vi "Load Transient.vi"() -> ()   [LabVIEW 2021]
uses:
  pmbus_ltm4676a/controls/ltm4676a_config.ctl
  controls/lt_nightwing_config.ctl
  controls/lt_heatwave_config.ctl
  controls/lt_system_timing_config.ctl
  <instrlib>/niDCPower/nidcpower.llb/niDCPower Source Mode.ctl
  <instrlib>/niDCPower/nidcpower.llb/niDCPower Output Function.ctl
  <instrlib>/niDCPower/nidcpower.llb/niDCPower Sense.ctl
  <instrlib>/niDCPower/nidcpower.llb/niDCPower Wait For Event - Event.ctl
  <instrlib>/niDCPower/nidcpower.llb/niDCPower Aperture Time Units.ctl
  <instrlib>/niDCPower/nidcpower.llb/niDCPower Export Signal - Signal.ctl
  <instrlib>/niDCPower/nidcpower.llb/niDCPower Disable Source Trigger With Channels.vi
panel:
  in  "App control":enum32{"Main", "Debug"}(tab)
  out "Load Transient Response":T1
  in  "Config control":T2(tab)
  in  "Source config":T3={"Source device name"="PXIe-4151", "Source device channel"="0", "Source device max. power (W)"=300.0, "Source device voltage (V)"=12.0, "Voltage GBW (Hz)"=2000.0, "Voltage comp. freq. (Hz)"=3530.0, "Voltage PZ ratio"=2.0}
  in  "Load config":T4={"Load device name"="PXIe-4051", "Load device channel"="0", "Load voltage limit (V)"=6.0, "Load device sample rate (S/s)"=1800000.0, "Current Setpoints"=[1.0, 20.0, 1.0], "Current GBW (Hz)"=14000.0, "Current comp. freq. (Hz)"=180000.0, "Current PZ ratio"=0.3} {"Current PZ ratio" min=0.0 max=8.0 step=0.1; "Current GBW (Hz)" min=0.0 step=1000.0; "Current Setpoints" format="%.2p"}
  in  "System timing config":T5={"DUT setup time (s)"=1.0, "Level dwell time (s)"=0.001, "Timeout (s)"=5.0} {"Timeout (s)" format="%.3p"; "Level dwell time (s)" step=0.0001; "DUT setup time (s)" format="%_4p"}
  in  "LTM4676A Runtime Config":T6={"SDC config path"=path "C:/dev/users/qkocian/opp_support/demos/argus-buck-demo/instrumentstudio/sdc/pmbus_ltm4676a.sdconfig", "Output setpoint (V)"=3.3, "Voltage margin (%)"=5.0, "Voltage warn limit (%)"=7.5, "Voltage fault limit (%)"=10.0, "Switching frequency (kHz)"=650} {"Switching frequency (kHz)" items=["250"=62440, "350"=64188, "425"=64338, "500"=64488, "575"=575, "650"=650, "750"=750, "1000"=1000]; "Voltage fault limit (%)" min=0.0 max=100.0 step=1.0 format="%.1g"; "Voltage warn limit (%)" min=0.0 max=100.0 step=1.0 format="%.1g"; "Voltage margin (%)" min=0.0 max=100.0 step=1.0 format="%.1g"; "Output setpoint (V)" min=0.5 max=5.5 step=0.1}
  in  "stop":bool
  out "success?":bool
  out "Current GBW readback (Hz)":dbl
  out "Current comp. freq. readback (Hz)":dbl
  out "Current PZ ratio readback":dbl
  in  "Waveform averages":i32=1
  out "Voltage GBW readback (Hz)":dbl
  out "Voltage comp. freq. readback (Hz)":dbl
  out "Voltage PZ ratio readback":dbl
  in  "Use PMBus?":bool
  # "Load SourceAdapt Readback"
  # "Source SourceAdapt Readback"
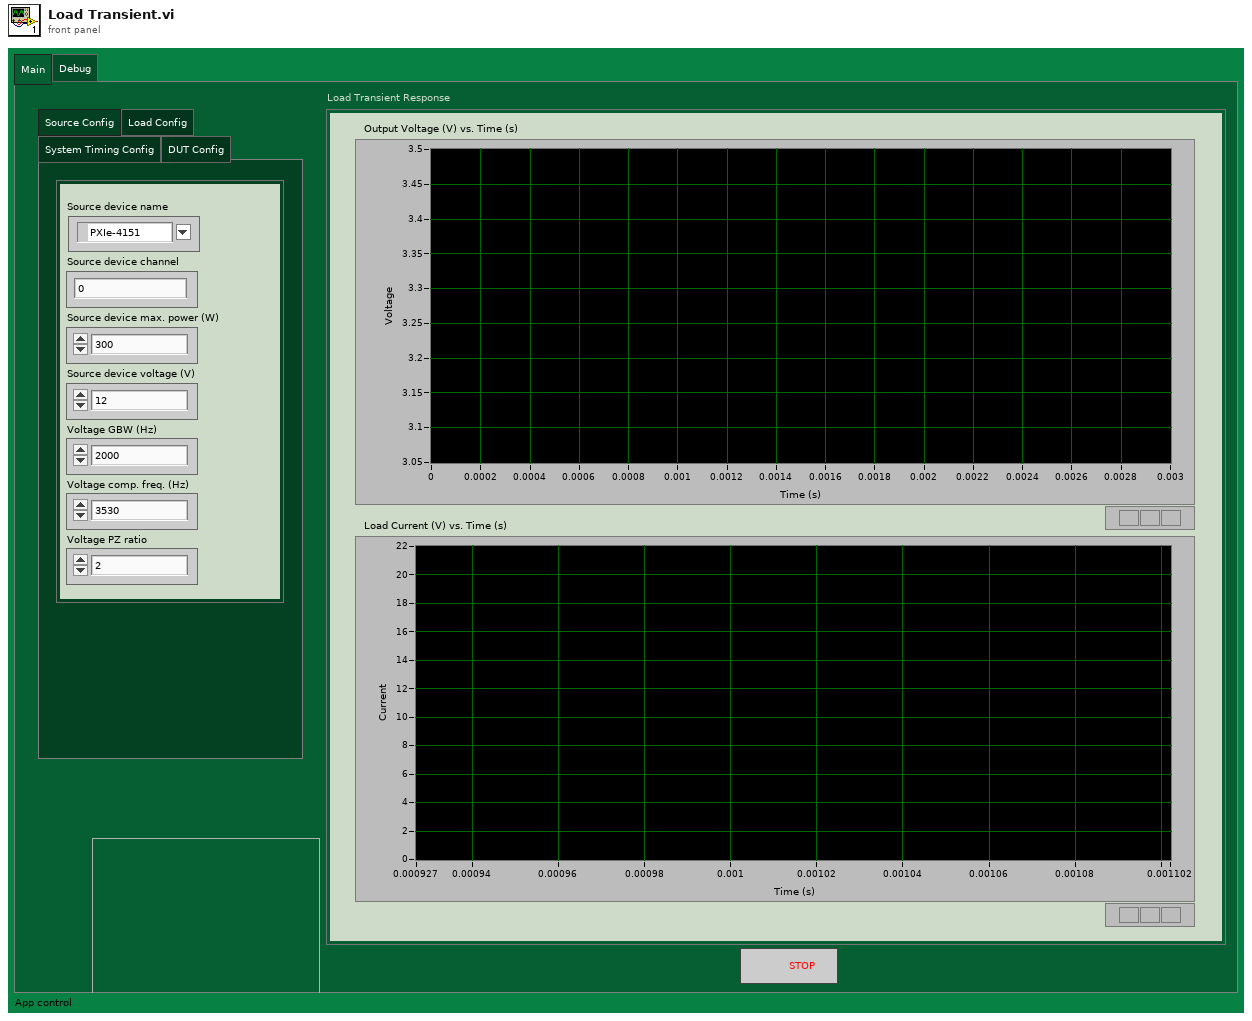
[diagram p1: front panel]
types:
  T1 = cluster{"Output Voltage (V) vs. Time (s)":waveform(dbl), "Load Current (V) vs. Time (s)":waveform(dbl)}
  T2 = enum32{"Source Config", "Load Config", "System Timing Config", "DUT Config"}
  T3 = typedef "lt_nightwing_config.ctl" = cluster{"Source device name":refnum<k15>, "Source device channel":string, "Source device max. power (W)":dbl, "Source device voltage (V)":dbl, "Voltage GBW (Hz)":dbl, "Voltage comp. freq. (Hz)":dbl, "Voltage PZ ratio":dbl}
  T4 = typedef "lt_heatwave_config.ctl" = cluster{"Load device name":refnum<k15>, "Load device channel":string, "Load voltage limit (V)":dbl, "Load device sample rate (S/s)":dbl, "Current Setpoints":dbl[], "Current GBW (Hz)":dbl, "Current comp. freq. (Hz)":dbl, "Current PZ ratio":dbl}
  T5 = typedef "lt_system_timing_config.ctl" = cluster{"DUT setup time (s)":dbl, "Level dwell time (s)":dbl, "Timeout (s)":dbl}
  T6 = typedef "ltm4676a_config.ctl" = cluster{"SDC config path":path, "Output setpoint (V)":dbl, "Voltage margin (%)":dbl, "Voltage warn limit (%)":dbl, "Voltage fault limit (%)":dbl, "Switching frequency (kHz)":u16}
  T7 = typedef "niDCPower Sense.ctl" = i32
  T8 = typedef "niDCPower Output Function.ctl" = i32
  T9 = typedef "niDCPower Source Mode.ctl" = i32
  T10 = typedef "niDCPower Wait For Event - Event.ctl" = i32
  T11 = typedef "niDCPower Export Signal - Signal.ctl" = i32
  T12 = typedef "niDCPower Aperture Time Units.ctl" = i32
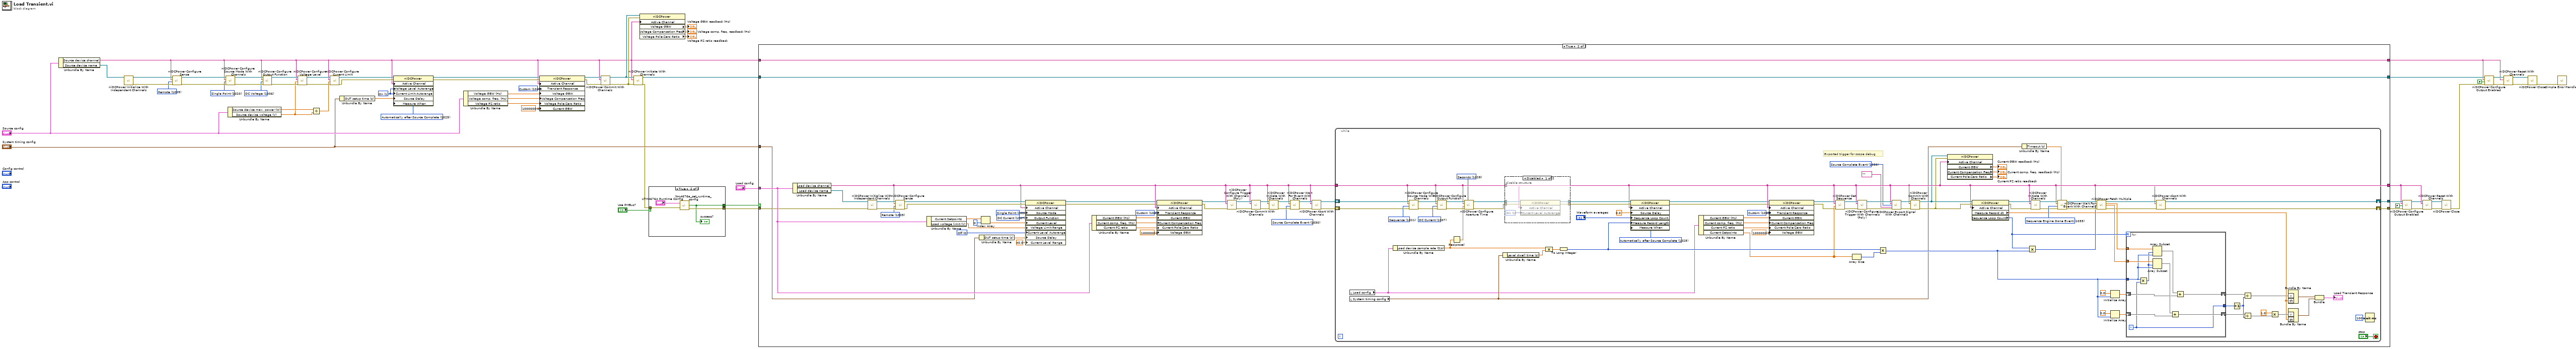
[diagram p0: block diagram]
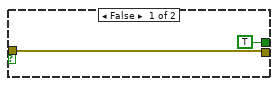
[diagram p2: hidden frame]
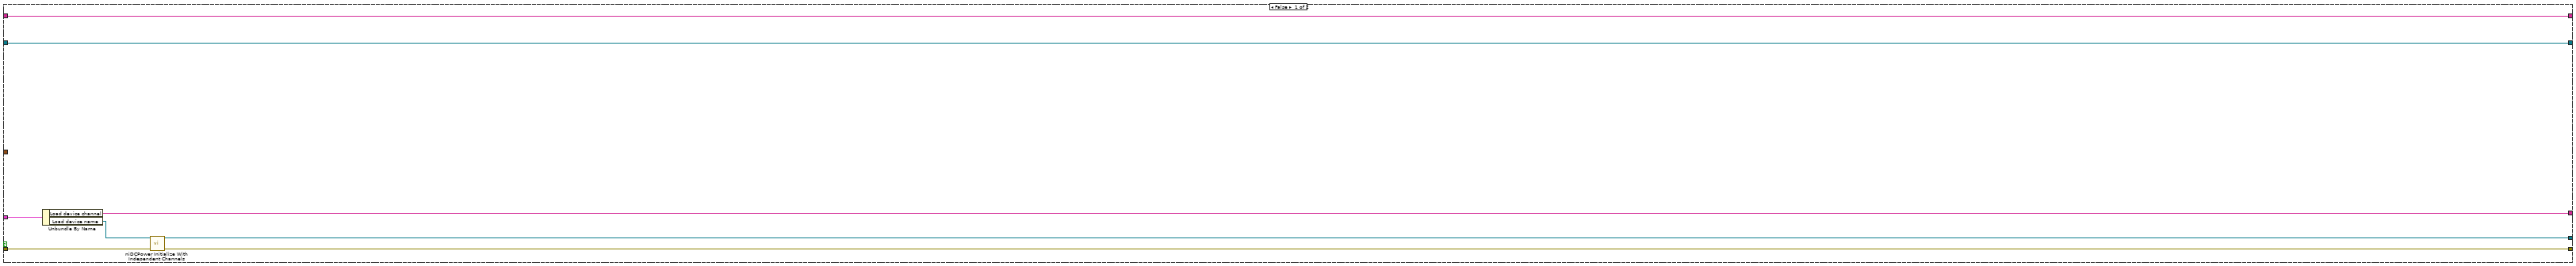
[diagram p3: hidden frame]
diagram:
  w32 = 1042 items=["Slow"=1041, "Normal"=1038, "Fast"=1039, "Custom"=1042] ("Source:Transient Response")
  w42 = T7 1009 items=["Local"=1008, "Remote"=1009] ("sense")
  w45 = 1025 items=["Automatically after Source Complete"=1025, "On Demand"=1026, "On Measure Trigger"=1027] ("Measurement:Advanced:Measure When")
  w54 = 1 items=["Off", "On"] ("Source:DC Voltage:Current Limit Autorange")
  w57 = T8 1006 items=["DC Voltage"=1006, "DC Current"=1007, "Pulse Voltage"=1049, "Pulse Current"=1050] ("output function")
  w60 = T9 1020 items=["Single Point"=1020, "Sequence"=1021] ("source mode")
  n1 = Unbundle By Name("Source config") -> ("Source device channel"=w3:string, "Source device name"=w30:refnum<k15>)
  n2 = call <instrlib>:"niDCPower Initialize With Independent Channels.vi"("resource name"=w30) -> ("error out"=w43:errorcluster, "instrument handle out"=w44:refnum<k15>)  [unwired: 9 in]
  n3 = call <instrlib>:"niDCPower Configure Sense.vi"("error in (no error)"=w43, "sense"=w42, "channel name"=w3, "instrument handle"=w44) -> ("error out"=w20:errorcluster, "instrument handle out"=w19:refnum<k15>)  [unwired: 6 in]
  n4 = call <instrlib>:"niDCPower Configure Source Mode With Channels.vi"("error in (no error)"=w20, "source mode"=w60, "channel name"=w3, "instrument handle"=w19) -> ("error out"=w59:errorcluster, "instrument handle out"=w58:refnum<k15>)  [unwired: 6 in]
  n5 = Unbundle By Name("Source config") -> ("Source device max. power (W)"=w29:dbl, "Source device voltage (V)"=w28:dbl)
  n6 = call <instrlib>:"niDCPower Configure Output Function.vi"("error in (no error)"=w59, "output function"=w57, "channel name"=w3, "instrument handle"=w58) -> ("error out"=w49:errorcluster, "instrument handle out"=w48:refnum<k15>)  [unwired: 6 in]
  n7 = call <instrlib>:"niDCPower Configure Voltage Level.vi"("error in (no error)"=w49, "voltage level"=w28, "channel name"=w3, "instrument handle"=w48) -> ("error out"=w46:errorcluster, "instrument handle out"=w47:refnum<k15>)  [unwired: 6 in]
  n8 = Divide(x=w29, y=w28) -> (x/y=w56:dbl)
  n9 = call <instrlib>:"niDCPower Configure Current Limit.vi"("error in (no error)"=w46, "current limit"=w56, "channel name"=w3, "instrument handle"=w47) -> ("error out"=w55:errorcluster, "instrument handle out"=w53:refnum<k15>)  [unwired: 6 in]
  n10 = Unbundle By Name("System timing config") -> ("DUT setup time (s)"=w23:dbl)
  n11 = property class="niDCPower"(reference=w53, error in=w55, "Active Channel"=w3, "Voltage Level Autorange"=w54, "Current Limit Autorange"=w54, "Source Delay"=w23, "Measure When"=w45) -> (reference out=w36:refnum<k15>, error out=w35:errorcluster)
  n12 = Unbundle By Name("Source config") -> ("Voltage GBW (Hz)"=w27:dbl, "Voltage comp. freq. (Hz)"=w26:dbl, "Voltage PZ ratio"=w25:dbl)
  n13 = property class="niDCPower"(reference=w36, error in=w35, "Active Channel"=w3, "Transient Response"=w32, "Voltage GBW"=w27, "Voltage Compensation Freq"=w26, "Voltage Pole-Zero Ratio"=w25, "Current GBW"=1000000.0 ("Source:Custom Transient Response:Current:Gain Bandwidth")) -> (reference out=w34:refnum<k15>, error out=w33:errorcluster)
  n14 = call <instrlib>:"niDCPower Commit With Channels.vi"("error in (no error)"=w33, "channel name"=w3, "instrument handle"=w34) -> ("error out"=w40:errorcluster, "instrument handle out"=w41:refnum<k15>)  [unwired: 7 in]
  n15 = call <instrlib>:"niDCPower Initiate With Channels.vi"("error in (no error)"=w40, "channel name"=w3, "instrument handle"=w41) -> ("error out"=w17:errorcluster, "instrument handle out"=w5:refnum<k15>)  [unwired: 7 in]
  n16 = property class="niDCPower"(reference=w41, error in=w40, "Active Channel"=w3) -> ("Voltage GBW"=→"Voltage GBW readback (Hz)":dbl, "Voltage Compensation Freq"=→"Voltage comp. freq. readback (Hz)":dbl, "Voltage Pole-Zero Ratio"=→"Voltage PZ ratio readback":dbl)  [unwired: 2 out]
  n17 = case shown="True" "Use PMBus?" {
    tunnel: [w64 w68] -> w18
    tunnel: w17 -> [w64 w67]
    tunnel: [TRUE ("success?") w65] -> w6
    frame False {
    }
    frame True {
      n18 = call "ltm4676a_set_runtime_config.vi"("LTM4676A Runtime Config"="LTM4676A Runtime Config", "error in (no error)"=w67) -> ("success?"=w65:bool, "error out"=w68:errorcluster)  [unwired: 1 out]
      "success?" <- w65
    }
  }
  n19 = case shown="True" w6 {
    tunnel: "Load config" -> [w75 w91]
    tunnel: "System timing config" -> [_ w90]
    tunnel: w18 -> [w71 w89]
    tunnel: [w69 w88] -> w16
    tunnel: [w71 w87] -> w15
    tunnel: [w74 w84] -> w14
    tunnel: w5 -> [w73 w85]
    tunnel: [w73 w85] -> w4
    tunnel: w3 -> [w72 w86]
    tunnel: [w72 w86] -> w2
    frame False {
      n20 = Unbundle By Name(w75) -> ("Load device channel"=w74:string, "Load device name"=w70:refnum<k15>)
      n21 = call <instrlib>:"niDCPower Initialize With Independent Channels.vi"("error in (no error)"=w71, "resource name"=w70) -> ("instrument handle out"=w69:refnum<k15>)  [unwired: 8 in, 1 out]
    }
    frame True {
      w79 = 0 items=["Off", "On"] ("Source:DC Current:Current Level Autorange")
      w98 = 1042 items=["Slow"=1041, "Normal"=1038, "Fast"=1039, "Custom"=1042] ("Source:Transient Response")
      w111 = T10 1030 items=["Source Complete Event"=1030, "Measure Complete Event"=1031, "Sequence Iteration Complete Event"=1032, "Sequence Engine Done Event"=1033, "Pulse Complete Event"=1051, "Ready For Pulse Trigger Event"=1052] ("event")
      w114 = 1007 items=["DC Voltage"=1006, "DC Current"=1007, "Pulse Voltage"=1049, "Pulse Current"=1050] ("Source:Output Function")
      w115 = 1020 items=["Single Point"=1020, "Sequence"=1021] ("Source:Source Mode")
      w116 = T7 1009 items=["Local"=1008, "Remote"=1009] ("sense")
      n22 = Unbundle By Name(w91) -> ("Load device channel"=w84:string, "Load device name"=w96:refnum<k15>)
      n23 = call <instrlib>:"niDCPower Initialize With Independent Channels.vi"("error in (no error)"=w89, "resource name"=w96) -> ("error out"=w118:errorcluster, "instrument handle out"=w117:refnum<k15>)  [unwired: 8 in]
      n24 = call <instrlib>:"niDCPower Configure Sense.vi"("error in (no error)"=w118, "sense"=w116, "channel name"=w84, "instrument handle"=w117) -> ("error out"=w107:errorcluster, "instrument handle out"=w108:refnum<k15>)  [unwired: 6 in]
      n25 = Unbundle By Name(w91) -> ("Current Setpoints"=w95:dbl[], "Load voltage limit (V)"=w76:dbl)
      n26 = Unbundle By Name(w90) -> ("DUT setup time (s)"=w97:dbl)
      n27 = Index Array(array=w95, index=0) -> (element=w105:dbl)
      n28 = property class="niDCPower"(reference=w108, error in=w107, "Active Channel"=w84, "Source Mode"=w115, "Output Function"=w114, "Current Level"=w105, "Voltage Limit Range"=w76, "Current Level Autorange"=w79, "Source Delay"=w97, "Current Level Range"=40.0 ("Source:DC Current:Current Level Range")) -> (reference out=w83:refnum<k15>, error out=w82:errorcluster)
      n29 = Unbundle By Name(w91) -> ("Current GBW (Hz)"=w94:dbl, "Current comp. freq. (Hz)"=w93:dbl, "Current PZ ratio"=w92:dbl)
      n30 = property class="niDCPower"(reference=w83, error in=w82, "Active Channel"=w84, "Transient Response"=w98, "Current GBW"=w94, "Current Compensation Freq"=w93, "Current Pole-Zero Ratio"=w92, "Voltage GBW"=1000000.0 ("Source:Custom Transient Response:Voltage:Gain Bandwidth")) -> (reference out=w81:refnum<k15>, error out=w80:errorcluster)
      n31 = call-poly <instrlib>:"niDCPower Configure Trigger With Channels (Poly).vi"("error in (no error)"=w80, "channel name"=w84, "instrument handle"=w81) -> ("error out"=w99:errorcluster, "instrument handle out"=w100:refnum<k15>)  [unwired: 7 in]
      n32 = call <instrlib>:"niDCPower Commit With Channels.vi"("error in (no error)"=w99, "channel name"=w84, "instrument handle"=w100) -> ("error out"=w101:errorcluster, "instrument handle out"=w102:refnum<k15>)  [unwired: 7 in]
      n33 = call <instrlib>:"niDCPower Initiate With Channels.vi"("error in (no error)"=w101, "channel name"=w84, "instrument handle"=w102) -> ("error out"=w113:errorcluster, "instrument handle out"=w112:refnum<k15>)  [unwired: 7 in]
      n34 = call <instrlib>:"niDCPower Wait For Event With Channels.vi"("error in (no error)"=w113, "event"=w111, "channel name"=w84, "instrument handle"=w112) -> ("error out"=w110:errorcluster, "instrument handle out"=w109:refnum<k15>)  [unwired: 6 in]
      n35 = call <instrlib>:"niDCPower Abort With Channels.vi"("error in (no error)"=w110, "channel name"=w84, "instrument handle"=w109) -> ("error out"=w103:errorcluster, "instrument handle out"=w104:refnum<k15>)  [unwired: 7 in]
      n36 = while {
        tunnel: w84 -> [w126]
        shift-right: [w137] -> w88
        shift-left: w104 -> [w180]
        shift-right: [w136] -> w87
        shift-left: w103 -> [w179]
        stop <- "stop" stop-if-true
        w131 = 1042 items=["Slow"=1041, "Normal"=1038, "Fast"=1039, "Custom"=1042] ("Source:Transient Response")
        w148 = T11 1030 items=["Source Complete Event"=1030, "Measure Complete Event"=1031, "Sequence Iteration Complete Event"=1032, "Sequence Engine Done Event"=1033, "Pulse Complete Event"=1051, "Ready For Pulse Trigger Event"=1052, "Start Trigger"=1034, "Source Trigger"=1035, "Measure Trigger"=1036, "Sequence Advance Trigger"=1037, "Pulse Trigger"=1053] ("signal")
        w144 = 1025 items=["Automatically after Source Complete"=1025, "On Demand"=1026, "On Measure Trigger"=1027] ("Measurement:Advanced:Measure When")
        w185 = T12 1028 items=["Seconds"=1028, "Powerline Cycles"=1029] ("aperture time units")
        w190 = T8 1007 items=["DC Voltage"=1006, "DC Current"=1007, "Pulse Voltage"=1049, "Pulse Current"=1050] ("output function")
        w199 = T10 1033 items=["Source Complete Event"=1030, "Measure Complete Event"=1031, "Sequence Iteration Complete Event"=1032, "Sequence Engine Done Event"=1033, "Pulse Complete Event"=1051, "Ready For Pulse Trigger Event"=1052] ("event")
        w201 = T9 1021 items=["Single Point"=1020, "Sequence"=1021] ("source mode")
        # "Exported trigger for scope debug"
        n37 = local read "Load config"() -> (w119:T4)
        n38 = local read "System timing config"() -> (w120:T5)
        n39 = Unbundle By Name(w119) -> ("Load device sample rate (S/s)"=w145:dbl)
        n40 = call <instrlib>:"niDCPower Configure Source Mode With Channels.vi"("error in (no error)"=w179, "source mode"=w201, "channel name"=w126, "instrument handle"=w180) -> ("error out"=w188:errorcluster, "instrument handle out"=w189:refnum<k15>)  [unwired: 6 in]
        n41 = call <instrlib>:"niDCPower Configure Output Function.vi"("error in (no error)"=w188, "output function"=w190, "channel name"=w126, "instrument handle"=w189) -> ("error out"=w186:errorcluster, "instrument handle out"=w187:refnum<k15>)  [unwired: 6 in]
        n42 = Reciprocal(x=w145) -> (1/x=w181:dbl)
        n43 = call <instrlib>:"niDCPower Configure Aperture Time.vi"("aperture time units"=w185, "error in (no error)"=w186, "aperture time"=w181, "channel name"=w126, "instrument handle"=w187) -> ("error out"=w134:errorcluster, "instrument handle out"=w135:refnum<k15>)  [unwired: 5 in]
        n44 = Unbundle By Name(w120) -> ("Level dwell time (s)"=w146:dbl)
        n45 = disable-structure shown="Disabled" {
          disable-tunnel: w135 -> [w207 w209]
          disable-tunnel: w134 -> [w206 w208]
          disable-tunnel: [w205 w209] -> w184
          disable-tunnel: [w204 w208] -> w183
          disable-tunnel: w126 -> [w202 _]
          frame Disabled {
            w203 = 1 items=["Off", "On"] ("Source:DC Current:Current Level Autorange")
            n46 = property class="niDCPower"(reference=w207, error in=w206, "Active Channel"=w202, "Current Level Autorange"=w203) -> (reference out=w205:refnum<k15>, error out=w204:errorcluster)
          }
          frame Enabled {
          }
        }
        n47 = Compound Arithmetic op=MULTIPLY(w145, w146) -> (w167:dbl)
        n48 = To Long Integer(number=w167) -> (32bit integer=w142:i32)
        n49 = property class="niDCPower"(reference=w184, error in=w183, "Active Channel"=w126, "Source Delay"=0.0 ("Source:Advanced:Source Delay"), "Sequence Loop Count"="Waveform averages", "Measure Record Length"=w142, "Measure When"=w144) -> (reference out=w125:refnum<k15>, error out=w124:errorcluster)
        n50 = Unbundle By Name(w119) -> ("Current GBW (Hz)"=w130:dbl, "Current comp. freq. (Hz)"=w129:dbl, "Current PZ ratio"=w128:dbl, "Current Setpoints"=w123:dbl[])
        n51 = property class="niDCPower"(reference=w125, error in=w124, "Active Channel"=w126, "Transient Response"=w131, "Current GBW"=w130, "Current Compensation Freq"=w129, "Current Pole-Zero Ratio"=w128, "Voltage GBW"=1000000.0 ("Source:Custom Transient Response:Voltage:Gain Bandwidth")) -> (reference out=w122:refnum<k15>, error out=w121:errorcluster)
        n52 = call <instrlib>:"niDCPower Set Sequence.vi"("error in (no error)"=w121, "values"=w123, "channel name"=w126, "instrument handle"=w122) -> ("error out"=w177:errorcluster, "instrument handle out"=w178:refnum<k15>)  [unwired: 6 in]
        n53 = Array Size(array=w123) -> (size(s)=w172:i32)
        n54 = call-poly <instrlib>:"niDCPower Configure Trigger With Channels (Poly).vi"("error in (no error)"=w177, "channel name"=w126, "instrument handle"=w178) -> ("error out"=w151:errorcluster, "instrument handle out"=w152:refnum<k15>)  [unwired: 7 in]
        n55 = Multiply(x=w142, y=w172) -> (x*y=w164:i32)
        n56 = call <instrlib>:"niDCPower Export Signal With Channels.vi"("instrument handle"=w152, "channel name"=w126, "signal"=w148, "output terminal"=tag "", "error in (no error)"=w151) -> ("instrument handle out"=w149:refnum<k15>, "error out"=w150:errorcluster)  [unwired: 9 in]
        n57 = call <instrlib>:"niDCPower Commit With Channels.vi"("error in (no error)"=w150, "channel name"=w126, "instrument handle"=w149) -> ("error out"=w141:errorcluster, "instrument handle out"=w173:refnum<k15>)  [unwired: 7 in]
        n58 = property class="niDCPower"(reference=w173, error in=w141, "Active Channel"=w126) -> ("Current GBW"=→"Current GBW readback (Hz)":dbl, "Current Compensation Freq"=→"Current comp. freq. readback (Hz)":dbl, "Current Pole-Zero Ratio"=→"Current PZ ratio readback":dbl)  [unwired: 2 out]
        n59 = property class="niDCPower"(reference=w173, error in=w141, "Active Channel"=w126) -> (reference out=w193:refnum<k15>, error out=w200:errorcluster, "Measure Record dt"=w157:dbl, "Sequence Loop Count"=w170:i32)
        n60 = Unbundle By Name(w120) -> ("Timeout (s)"=w140:dbl)
        n61 = Multiply(x=w170, y=w164) -> (x*y=w171:i32)
        n62 = call <instrlib>:"niDCPower Initiate With Channels.vi"("error in (no error)"=w200, "channel name"=w126, "instrument handle"=w193) -> ("error out"=w153:errorcluster, "instrument handle out"=w154:refnum<k15>)  [unwired: 7 in]
        n63 = call <instrlib>:"niDCPower Wait For Event With Channels.vi"("timeout (10.0)"=w140, "error in (no error)"=w153, "event"=w199, "channel name"=w126, "instrument handle"=w154) -> ("error out"=w197:errorcluster, "instrument handle out"=w198:refnum<k15>)  [unwired: 5 in]
        n64 = call <instrlib>:"niDCPower Fetch Multiple.vi"("instrument handle"=w198, "channel name"=w126, "count (1)"=w171, "error in (no error)"=w197) -> ("instrument handle out"=w139:refnum<k15>, "voltage measurements"=w169:dbl[], "current measurements"=w168:dbl[], "error out"=w138:errorcluster)  [unwired: 6 in, 2 out]
        n65 = Initialize Array(0.0 ("element"), w164) -> (w163:dbl[])
        n66 = Initialize Array(0.0 ("element"), w164) -> (w162:dbl[])
        n67 = for {
          N: w170 -> [_]
          tunnel: w169 -> [w220]
          tunnel: w168 -> [w219]
          tunnel: w164 -> [w218]
          shift-right: [w212] -> w159
          shift-left: w162 -> [w213]
          shift-right: [w211] -> w160
          shift-left: w163 -> [w214]
          tunnel: [w210] -> w161
          i -> [w210]
          n68 = Multiply(x=w218, y=w210) -> (x*y=w217:i32)
          n69 = Array Subset(array=w220, index=w217, length=w218) -> (w216:dbl[])
          n70 = Array Subset(array=w219, index=w217, length=w218) -> (w215:dbl[])
          n71 = Add(x=w215, y=w213) -> (x+y=w212:dbl[])
          n72 = Add(x=w216, y=w214) -> (x+y=w211:dbl[])
        }
        n73 = call <instrlib>:"niDCPower Abort With Channels.vi"("error in (no error)"=w138, "channel name"=w126, "instrument handle"=w139) -> ("error out"=w136:errorcluster, "instrument handle out"=w137:refnum<k15>)  [unwired: 7 in]
        n74 = Increment(x=w161) -> (x+1=w158:i32)
        n75 = Divide(x=w160, y=w158) -> (x/y=w155:dbl[])
        n76 = Divide(x=w159, y=w158) -> (x/y=w156:dbl[])
        n77 = Multiply(x=1.0, y=w156) -> (x*y=w192:dbl[])
        n78 = Bundle By Name("Y"=w155, "dt"=w157) -> (w196:waveform(dbl))  [unwired: 1 in]
        n79 = Bundle By Name("Y"=w192, "dt"=w157) -> (w195:waveform(dbl))  [unwired: 1 in]
        n80 = Bundle(w196, w195) -> (→"Load Transient Response":cluster{waveform(dbl), waveform(dbl)})  [unwired: 1 in]
        n81 = Wait (ms)(milliseconds to wait=u32 100) -> ()  [unwired: 1 out]
      }
    }
  }
  n82 = call <instrlib>:"niDCPower Configure Output Enabled.vi"("error in (no error)"=w15, "output enabled"=FALSE, "channel name"=w14, "instrument handle"=w16) -> ("error out"=w12:errorcluster, "instrument handle out"=w13:refnum<k15>)  [unwired: 6 in]
  n83 = call <instrlib>:"niDCPower Reset With Channels.vi"("error in (no error)"=w12, "channel name"=w14, "instrument handle"=w13) -> ("error out"=w62:errorcluster, "instrument handle out"=w61:refnum<k15>)  [unwired: 7 in]
  n84 = call <instrlib>:"niDCPower Close.vi"("error in (no error)"=w62, "instrument handle"=w61) -> ("error out"=w10:errorcluster)  [unwired: 9 in]
  n85 = call <instrlib>:"niDCPower Configure Output Enabled.vi"("error in (no error)"=w10, "output enabled"=FALSE, "channel name"=w2, "instrument handle"=w4) -> ("error out"=w7:errorcluster, "instrument handle out"=w8:refnum<k15>)  [unwired: 6 in]
  n86 = call <instrlib>:"niDCPower Reset With Channels.vi"("error in (no error)"=w7, "channel name"=w2, "instrument handle"=w8) -> ("error out"=w51:errorcluster, "instrument handle out"=w52:refnum<k15>)  [unwired: 7 in]
  n87 = call <instrlib>:"niDCPower Close.vi"("error in (no error)"=w51, "instrument handle"=w52) -> ("error out"=w50:errorcluster)  [unwired: 9 in]
  n88 = call <vilib>:"Simple Error Handler.vi"("error in (no error)"=w50) -> ()  [unwired: 4 in, 5 out]
